vi "ResetChartd.vi"(8 "error in (no error)":errorcluster, 9 "reference":refnum<vi>, 10 "Bottom":T1, 11 "Top":T1) -> (0 "error out":errorcluster)   [LabVIEW 2016]
uses:
  Typedefs/Hit chart cluster refnum.ctl
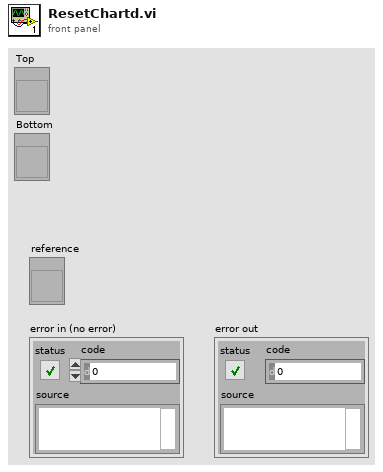
[diagram p1: front panel]
types:
  T1 = typedef "Hit chart cluster refnum.ctl" = refnum<vi>
  T2 = cluster{"Total hits":dbl, "Ratio":dbl, "Non-coincidences":dbl, "Coincidences":dbl}[]
  T3 = typedef "HitChart refnum.ctl" = refnum<vi>
  T4 = typedef "HitChart.ctl" = cluster{"Waveform Chart":cluster{"Coincidences":dbl, "Non-coincidences":dbl, "Ratio":dbl, "Total hits":dbl}[], "Last update timestamp":timestamp, "Resolution(s)":dbl, "nondisplayed coincs":i32, "nondisplayed noncoincs":i32, "Last upd":i64, "ID":i8}
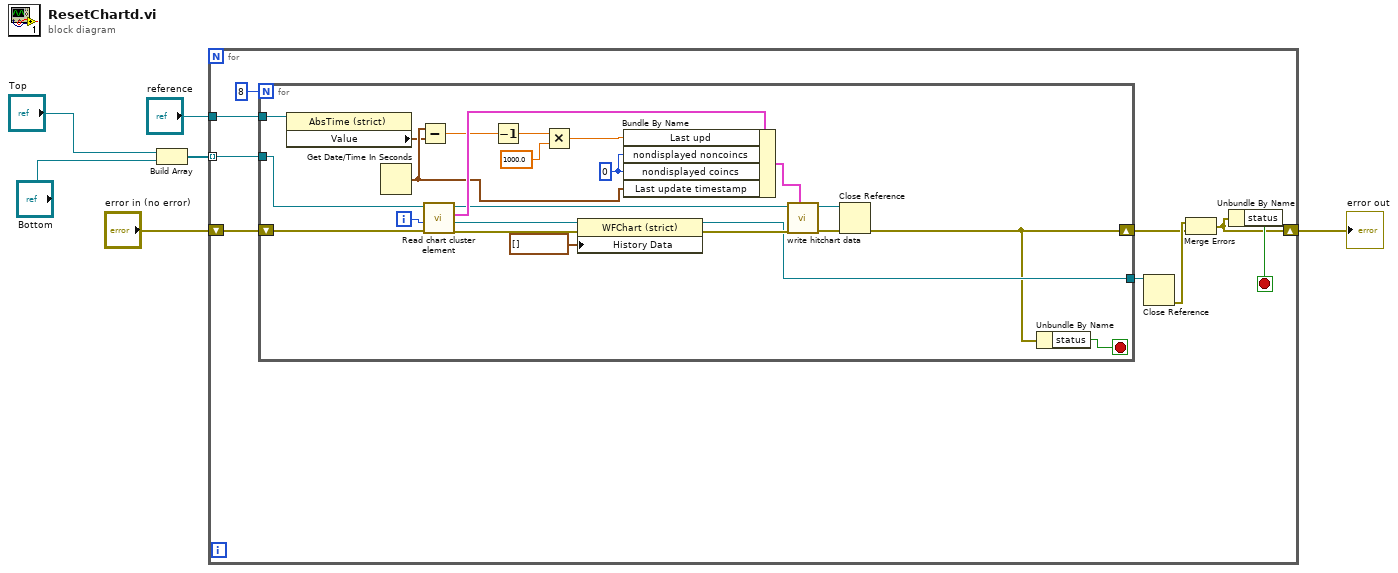
[diagram p0: block diagram]
diagram:
  n1 = Build Array("Top", "Bottom") -> (w4:T1[])
  n2 = for {
    tunnel: w4 -> [w14] mode=indexing
    shift-right: [w8] -> w6
    shift-left: "error in (no error)" -> [w12]
    tunnel: "reference" -> [w7]
    stop <- w11 stop-if-true
    n3 = for {
      N: 8 -> [_]
      shift-right: [w19] -> w9
      shift-left: w12 -> [w37]
      tunnel: w14 -> [w16]
      tunnel: [w20] -> w13
      tunnel: w7 -> [w26]
      i -> [w38]
      stop <- w18 stop-if-true
      w35 = 0 ("nondisplayed noncoincs")
      n4 = property class="AbsTime (strict)"(reference=w26) -> ("Value"=w33:timestamp)  [unwired: 1 in, 2 out]
      n5 = Get Date/Time In Seconds() -> (seconds since 1Jan1904=w34:timestamp)
      n6 = Subtract(x=w34, y=w33) -> (x-y=w31:dbl)
      n7 = call "Read chart cluster element.vi"("error in (no error)"=w37, "Chart cluster element"=w38, "Chart cluster"=w16) -> ("error out"=w23:errorcluster, "Chart ref"=w24:T3, 2:"Chart cluster"=w36:T4, 3:"Chart cluster"=w25:T1)  [unwired: 5 in]
      n8 = Decrement(x=w31) -> (x-1=w30:dbl)
      n9 = Multiply(x=w30, y=1000.0) -> (x*y=w17:dbl)
      n10 = property class="WFChart (strict)"(reference=w24, error in=w23, "History Data"=T2 []) -> (reference out=w20:T3, error out=w22:errorcluster)
      n11 = Bundle By Name(cluster=w36, "Last upd"=w17, "nondisplayed noncoincs"=w35, "nondisplayed coincs"=w35, "Last update timestamp"=w34) -> (w29:T4)
      n12 = call "write hitchart data.vi"("Histogram cluster"=w29, "error in (no error)"=w22, "Hit charts"=w25) -> ("error out"=w27:errorcluster, "Hit charts"=w28:T1)  [unwired: 7 in]
      n13 = Close Reference(reference=w28, error in (no error)=w27) -> (error out=w19:errorcluster)
      n14 = Unbundle By Name(w19) -> ("status"=w18:bool)
    }
    n15 = Close Reference(reference=w13) -> (error out=w10:errorcluster)  [unwired: 1 in]
    n16 = Merge Errors(w10, w9) -> (w8:errorcluster)
    n17 = Unbundle By Name(w8) -> ("status"=w11:bool)
  }
  "error out" <- w6
